vi "Configure A Trigger Mode.vi"(0 "VISA resource name":refnum<visa-resource-name>, 1 "Trigger Level Preference (0:Independent)":u16(ring) items=["Independent", "Shared"], 5 "Trigger Mode (0:Normal)":u16(ring) items=["Normal", "Auto"], 7 "Holdoff Type (0:Auto)":u16(ring) items=["Auto", "Time", "Random"], 9 "Time Holdoff (1us)":dbl=1e-06, 11 "error in (no error)":errorcluster) -> (4 "VISA resource name out":refnum<visa-resource-name>, 15 "error out":errorcluster)   [LabVIEW 2012, in "Tektronix 7000 Series.lvlib"]
doc: "Configures the A trigger mode of an oscilloscope. You can configure trigger mode, holdoff type, and trigger level preference only when you set trigger type to A trigger."
uses:
  Tektronix 7000 Series.lvlib
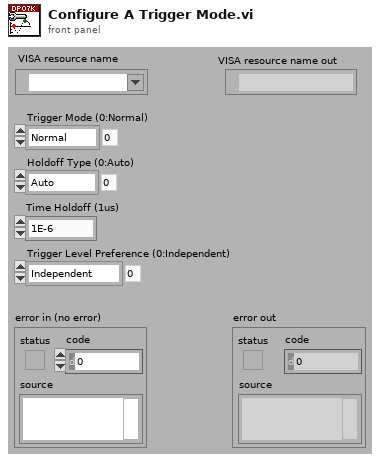
[diagram p1: front panel]
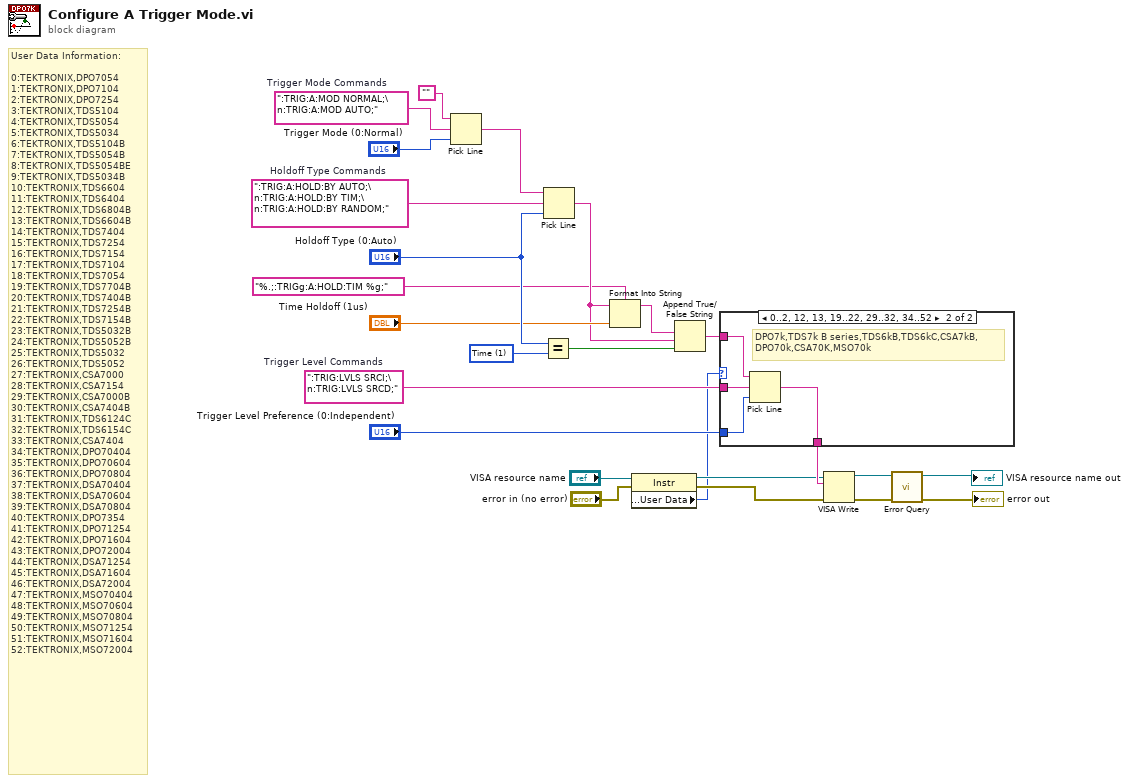
[diagram p0: block diagram]
diagram:
  w12 = ":TRIG:LVLS SRCI;\n:TRIG:LVLS SRCD;"  # Trigger Level Commands
  w20 = u16 1 items=["Auto", "Time", "Random", "Default"] ("Holdoff Type (0:Auto)")
  w21 = ":TRIG:A:HOLD:BY AUTO;\n:TRIG:A:HOLD:BY TIM;\n:TRIG:A:HOLD:BY RANDOM;"  # Holdoff Type Commands
  w25 = ":TRIG:A:MOD NORMAL;\n:TRIG:A:MOD AUTO;"  # Trigger Mode Commands
  # "User Data Information:\n\n0:TEKTRONIX,DPO7054\n1:TEKTRONIX,DPO7104\n2:TEKTRONIX,DPO7254\n3:TEKTRONIX,TDS5104\n4:TEKTRONIX,TDS5054\n5:TEKTRONIX,TDS5034\n6:TEKTRONIX,TDS5104B\n7:TEKTRONIX,TDS5054B\n8:TEKTRONIX,TDS5054BE\n9:TEKTRONIX,TDS5034B\n10:TEKTRONIX,TDS6604\n11:TEKTRONIX,TDS6404\n12:TEKTRONIX,TDS6804B\n13:TEKTRONIX,TDS6604B\n14:TEKTRONIX,TDS7404\n15:TEKTRONIX,TDS7254\n16:TEKTRONIX,TDS7154\n17:TEKTRONIX,TDS7104\n18:TEKTRONIX,TDS7054\n19:TEKTRONIX,TDS7704B\n20:TEKTRONIX,TDS7404B\n21:TEKTRONIX,TDS7254B\n22:TEKTRONIX,TDS7154B\n23:TEKTRONIX,TDS5032B\n24:TEKTRONIX,TDS5052B\n25:TEKTRONIX,TDS5032\n26:TEKTRONIX,TDS5052\n27:TEKTRONIX,CSA7000\n28:TEKTRONIX,CSA7154\n29:TEKTRONIX,CSA7000B\n30:TEKTRONIX,CSA7404B\n31:TEKTRONIX,TDS6124C\n32:TEKTRONIX,TDS6154C\n33:TEKTRONIX,CSA7404\n34:TEKTRONIX,DPO70404\n35:TEKTRONIX,DPO70604\n36:TEKTRONIX,DPO70804\n37:TEKTRONIX,DSA70404\n38:TEKTRONIX,DSA70604\n39:TEKTRONIX,DSA70804\n40:TEKTRONIX,DPO7354\n41:TEKTRONIX,DPO71254\n42:TEKTRONIX,DPO71604\n43:TEKTRONIX,DPO72004\n44:TEKTRONIX,DSA71254\n45:TEKTRONIX,DSA71604\n46:TEKTRONIX,DSA72004\n47:TEKTRONIX,MSO70404\n48:TEKTRONIX,MSO70604\n49:TEKTRONIX,MSO70804\n50:TEKTRONIX,MSO71254\n51:TEKTRONIX,MSO71604\n52:TEKTRONIX,MSO72004"
  n1 = Pick Line(string ("")="" ("Empty String Constant"), multi-line string=w25, line index="Trigger Mode (0:Normal)") -> (output string=w22:string)
  n2 = Equal?(x="Holdoff Type (0:Auto)", y=w20) -> (x = y?=w18:bool)
  n3 = Pick Line(string ("")=w22, multi-line string=w21, line index="Holdoff Type (0:Auto)") -> (output string=w15:string)
  n4 = Format Into String(format string="%.;:TRIGg:A:HOLD:TIM %g;", initial string=w15, "Time Holdoff (1us)") -> (resulting string=w16:string)  [unwired: 1 in, 1 out]
  n5 = property class="Instr"(reference="VISA resource name", error in="error in (no error)") -> (reference out=w6:refnum<visa-resource-name>, error out=w4:errorcluster, "General Settings:User Data"=w3:u32)
  n6 = Append True/False String(1:w18, 2:w15, 3:w16) -> (0:w13:string)  [unwired: 1 in]
  n7 = case shown="0..2, 12, 13, 19..22, 29..32, 34..52" w3 {
    tunnel: w13 -> [w26 w30]
    tunnel: w12 -> [_ w29]
    tunnel: "Trigger Level Preference (0:Independent)" -> [_ w28]
    tunnel: [w26 w27] -> w7
    frame Default {
    }
    frame 0..2, 12, 13, 19..22, 29..32, 34..52 {
      # "DPO7k,TDS7k B series,TDS6kB,TDS6kC,CSA7kB,\nDPO70k,CSA70K,MSO70k"
      n8 = Pick Line(string ("")=w30, multi-line string=w29, line index=w28) -> (output string=w27:string)
    }
  }
  n9 = VISA Write(VISA resource name=w6, write buffer=w7, error in (no error)=w4) -> (VISA resource name out=w9:refnum<visa-resource-name>, error out=w10:errorcluster)  [unwired: 1 out]
  n10 = call "Error Query.vi"("error in (no error)"=w10, "VISA resource name"=w9) -> ("error out"=→"error out":errorcluster, "VISA resource name out"=→"VISA resource name out":refnum<visa-resource-name>)  [unwired: 6 in, 2 out]
